vi "MissionLocation.vi"(8 "error in (no error)":errorcluster, 11 "RoundBouy in":refnum<class "RoundBouy.lvclass">) -> (0 "error out":errorcluster, 2 "bouy location":T1 {"North" format="%#_10f"; "East" format="%#_8f"}, 3 "RoundBouy out":refnum<class "RoundBouy.lvclass">)   [LabVIEW 2012, in "RoundBouy.lvclass"]
uses:
  RoundBouy.lvclass
  Data/TypeDefs/UTM Location.ctl
  RoundBouy.lvclass/RoundBouy.ctl
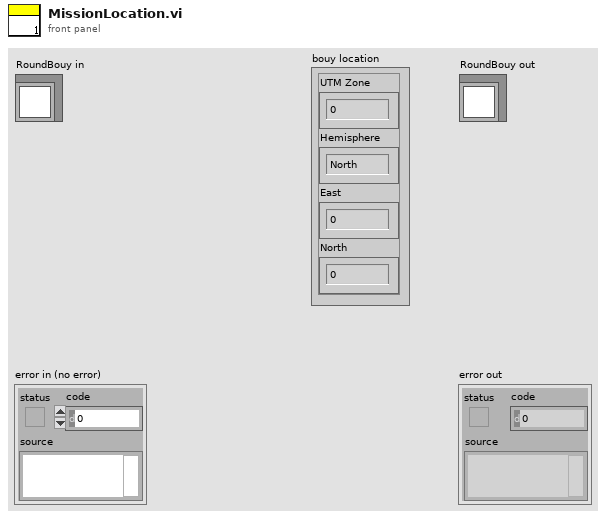
[diagram p1: front panel]
types:
  T1 = typedef "UTM Location.ctl" = cluster{"UTM Zone":dbl, "Hemisphere":enum16{"North", "South"}, "East":dbl, "North":dbl}
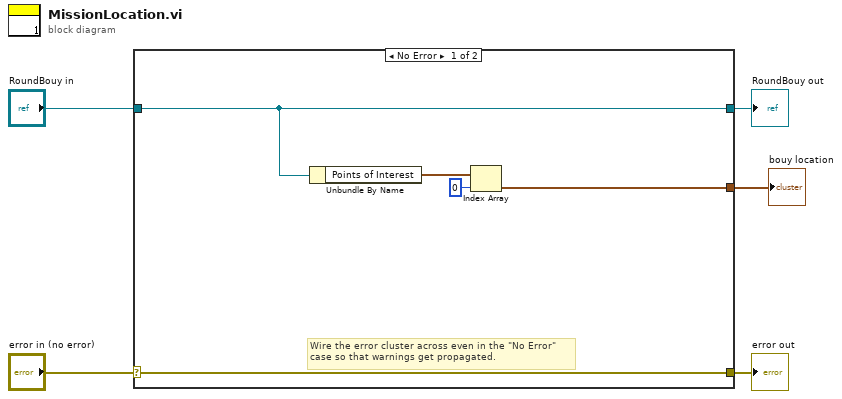
[diagram p0: block diagram]
diagram:
  n1 = case shown="No Error" "error in (no error)" {
    selector: "error in (no error)" -> [w10 w12]
    tunnel: [w10 w12] -> w4
    tunnel: [w9 w11] -> w2
    tunnel: "RoundBouy in" -> [w9 w11]
    tunnel: [w6 _] -> w1
    frame No Error {
      # "Wire the error cluster across even in the \"No Error\"\ncase so that warnings get propagated."
      n2 = Unbundle By Name(w9) -> ("Points of Interest"=w8:T1[])
      n3 = Index Array(array=w8, index=0) -> (element=w6:T1)
    }
    frame Error {
    }
  }
  "error out" <- w4
  "RoundBouy out" <- w2
  "bouy location" <- w1
